vi "FindConfPath.vi"(8 "error in":errorcluster, 9 "FileName":string="Configuration.ini", 10 "SubFolder":string="Configuration", 11 "Application in":refnum<vi>) -> (0 "error out":errorcluster, 3 "conf path":path)   [LabVIEW 2020]
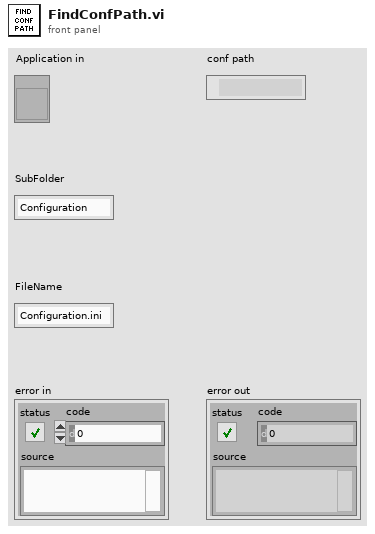
[diagram p1: front panel]
types:
  T1 = enum32{"invalid app kind", "Development System", "Run Time System", "Student Edition", "Embedded LabVIEW", "Evaluation", "Custom"}
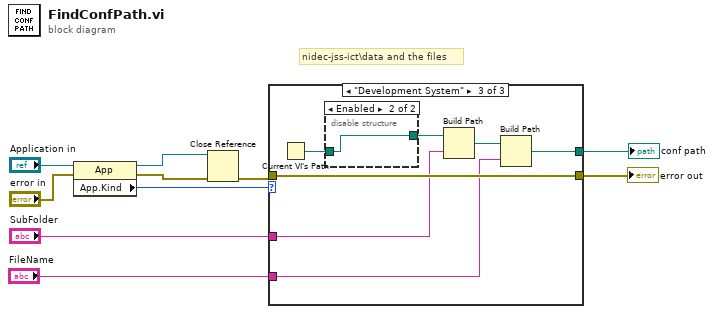
[diagram p0: block diagram]
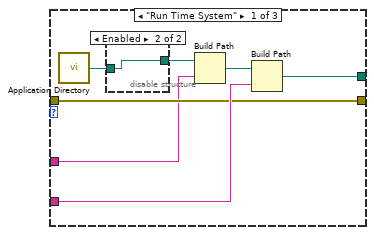
[diagram p2: hidden frame]
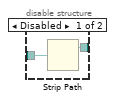
[diagram p3: hidden frame]
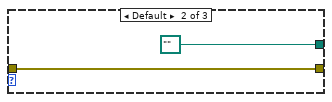
[diagram p4: hidden frame]
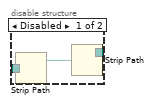
[diagram p5: hidden frame]
diagram:
  # "nidec-jss-ict\\data and the files"
  n1 = property class="App"(reference="Application in", error in="error in") -> (reference out=w10:refnum<vi>, error out=w9:errorcluster, "App.Kind"=w7:T1)
  n2 = Close Reference(reference=w10, error in (no error)=w9) -> (error out=w8:errorcluster)
  n3 = case shown="\"Development System\"" w7 {
    tunnel: w8 -> [w15 w21 w29]
    tunnel: "FileName" -> [w16 _ w23]
    tunnel: [w15 w21 w29] -> w3
    tunnel: [w14 path "" ("appended path") w24] -> w1
    tunnel: "SubFolder" -> [w13 _ w25]
    frame "Run Time System" {
      n4 = call <vilib>:"Application Directory.vi"() -> ("Application Directory"=w12:path)
      n5 = disable-structure shown="Enabled" {
        disable-tunnel: w12 -> [w19 w20]
        disable-tunnel: [w18 w20] -> w11
        frame Disabled {
          n6 = Strip Path(path=w19) -> (stripped path=w18:path)  [unwired: 1 out]
        }
        frame Enabled {
        }
      }
      n7 = Build Path(base path=w11, name or relative path=w13) -> (appended path=w17:path)
      n8 = Build Path(base path=w17, name or relative path=w16) -> (appended path=w14:path)
    }
    frame Default {
    }
    frame "Development System" {
      n9 = Current VI's Path() -> (path=w26:path)
      n10 = disable-structure shown="Enabled" {
        disable-tunnel: [w32 w33] -> w28
        disable-tunnel: w26 -> [w31 w33]
        frame Disabled {
          n11 = Strip Path(path=w31) -> (stripped path=w30:path)  [unwired: 1 out]
          n12 = Strip Path(path=w30) -> (stripped path=w32:path)  [unwired: 1 out]
        }
        frame Enabled {
        }
      }
      n13 = Build Path(base path=w28, name or relative path=w25) -> (appended path=w27:path)
      n14 = Build Path(base path=w27, name or relative path=w23) -> (appended path=w24:path)
    }
  }
  "conf path" <- w1
  "error out" <- w3
